vi "Create.vi"(5 "response (type)":refnum<class "response.lvclass">, 8 "error in (no error)":errorcluster, 9 "body":string, 10 "headers":string) -> (0 "error out":errorcluster, 3 "response out":refnum<class "response.lvclass">)   [LabVIEW 2020, in "http.lvlib" / "response.lvclass"]
uses:
  response.lvclass
  response.lvclass/response.ctl
  Response Headers/Response Headers.lvclass
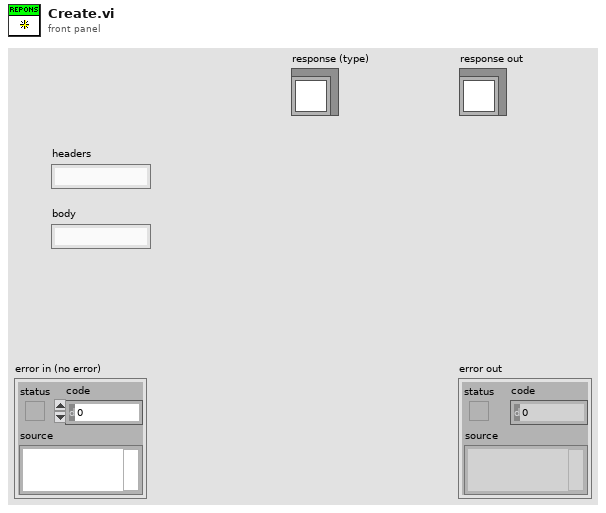
[diagram p1: front panel]
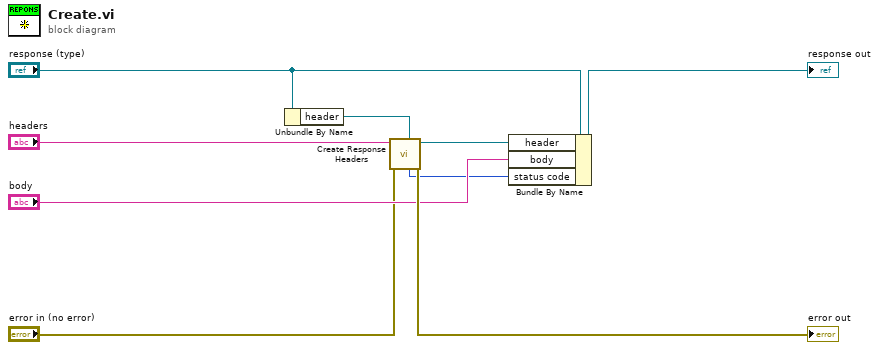
[diagram p0: block diagram]
diagram:
  n1 = Unbundle By Name("response (type)") -> ("header"=w3:refnum<class "Response Headers.lvclass">)
  n2 = call "Create Response Headers.vi"("Response Headers in"=w3, "error in (no error)"="error in (no error)", "Response Headers"="headers") -> ("error out"=→"error out":errorcluster, "Response Headers out"=w4:refnum<class "Response Headers.lvclass">, "status code"=w2:u16)  [unwired: 6 in]
  n3 = Bundle By Name(cluster="response (type)", "header"=w4, "body"="body", "status code"=w2) -> (→"response out":refnum<class "response.lvclass">)
